vi "MT Generate Bits (poly).vi"   [LabVIEW 2020, in "niDMT.lvlib"]
doc: "Generates the sequence of data bits to be modulated. This polymorphic VI can generate Fibonacci or Galois pseudonoise (PN) bit sequences. The VI can also generate bit sequences based on a pattern that you specify. The VI repeats the selected pattern until it generates the number of bits that you specify in the <B>total bits</B>."
uses:
  <vilib>/addons/Modulation/niDMT.lvlib
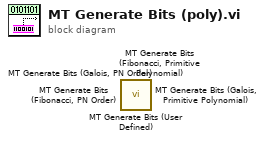
[diagram p0: block diagram]
diagram:
  n1 = call <vilib>:"MT Generate Bits (User Defined).vi"() -> ()  [unwired: 14 in, 2 out]
  n2 = call <vilib>:"MT Generate Bits (Fibonacci, Primitive Polynomial).vi"() -> ()  [unwired: 13 in, 3 out]
  n3 = call <vilib>:"MT Generate Bits (Fibonacci, PN Order).vi"() -> ()  [unwired: 13 in, 3 out]
  n4 = call <vilib>:"MT Generate Bits (Galois, Primitive Polynomial).vi"() -> ()  [unwired: 13 in, 3 out]
  n5 = call <vilib>:"MT Generate Bits (Galois, PN Order).vi"() -> ()  [unwired: 13 in, 3 out]
